vi "CheckFuncInstr.vi"(8 "error in (no error)":errorcluster caption="entrée d'erreur (pas d'erreur)", 11 "Experiment en entrée":refnum<class "Experiment.lvclass"> caption="DNL_LabVIEW Object in") -> (0 "error out":errorcluster caption="sortie d'erreur", 3 "Experiment en sortie":refnum<class "Experiment.lvclass"> caption="DNL_LabVIEW Object out")   [LabVIEW 2019, in "Experiment.lvclass"]
uses:
  Experiment.lvclass
  Experiment.lvclass/Experiment.ctl
  DevicesClass/BaseDevice/BaseDevice.lvclass
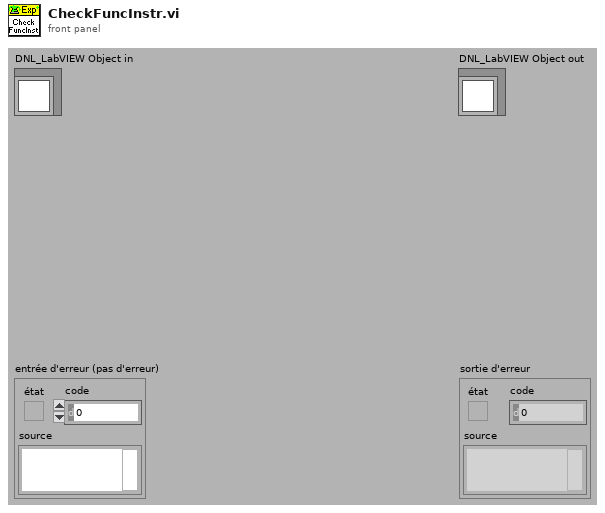
[diagram p1: front panel]
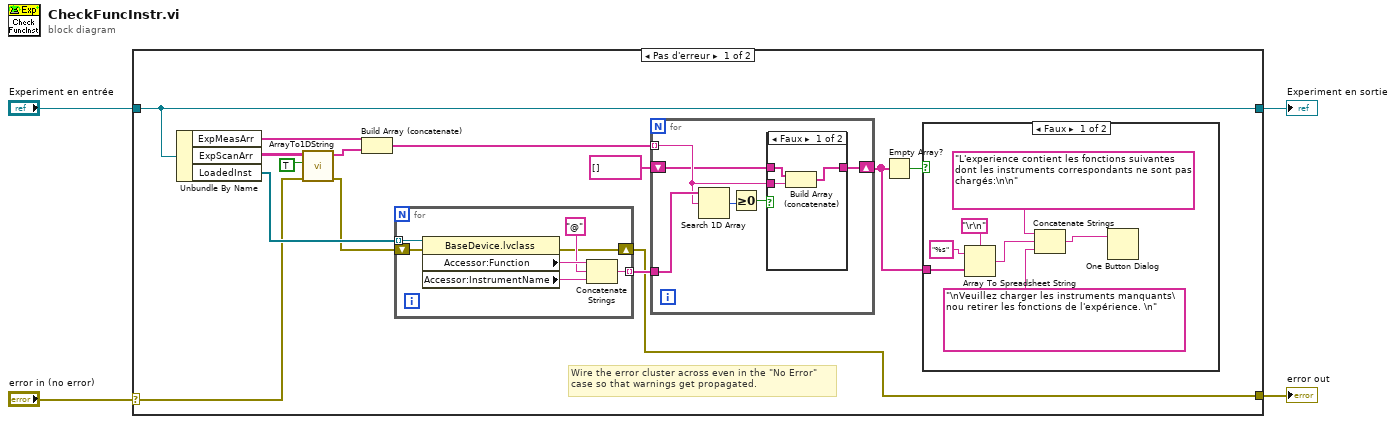
[diagram p0: block diagram]
diagram:
  n1 = case shown="Pas d'erreur" "error in (no error)" {
    selector: "error in (no error)" -> [w10 w44]
    tunnel: [w6 w44] -> w3
    tunnel: [w18 w43] -> w1
    tunnel: "Experiment en entrée" -> [w18 w43]
    frame No Error {
      # "Wire the error cluster across even in the \"No Error\"\ncase so that warnings get propagated."
      n2 = Unbundle By Name(w18) -> ("ExpMeasArr"=w16:string[], "ExpScanArr"=w14:string[][], "LoadedInst"=w17:refnum<class "BaseDevice.lvclass">[])
      n3 = call <userlib>:"ArrayTo1DString.vi"("ErrorIn(No Error)"=w10, "DelArrEnd(F)"=TRUE ("DelArrEnd"), "tableau"=w14) -> ("sortie d'erreur"=w9:errorcluster, "Array Out"=w13:string[])  [unwired: 6 in, 1 out]
      n4 = Build Array (concatenate)(w16, w13) -> (w15:string[])
      n5 = for {
        tunnel: w17 -> [w32] mode=indexing
        tunnel: [w28] -> w11 mode=indexing
        shift-right: [w27] -> w6
        shift-left: w9 -> [w26]
        n6 = property class="BaseDevice.lvclass"(reference=w32, error in=w26) -> (error out=w27:errorcluster, "Accessor:Function"=w31:string, "Accessor:InstrumentName"=w30:string)  [unwired: 1 out]
        n7 = Concatenate Strings(w31, "@" ("chaîne"), w30) -> (w28:string)
      }
      n8 = for {
        tunnel: w15 -> [w34] mode=indexing
        tunnel: w11 -> [w38]
        shift-right: [w35] -> w7
        shift-left: string[] [] -> [w33]
        n9 = Search 1D Array(1D array=w38, element=w34) -> (index of element=w37:i32)  [unwired: 1 in]
        n10 = Greater Or Equal To 0?(x=w37) -> (x >= 0?=w36:bool)
        n11 = case shown="Faux" w36 {
          tunnel: [w40 w42] -> w35
          tunnel: w34 -> [w41 _]
          tunnel: w33 -> [w39 w42]
          frame False {
            n12 = Build Array (concatenate)(w39, w41) -> (w40:string[])
          }
          frame True {
          }
        }
      }
      n13 = Empty Array?(array=w7) -> (empty?=w8:bool)
      n14 = case shown="Faux" w8 {
        tunnel: w7 -> [w25 _]
        frame False {
          n15 = Array To Spreadsheet String(delimiter (Tab)="\r\n", array=w25, 3:"%s" ("séparateur (Tabulation)")) -> (spreadsheet string=w22:string)
          n16 = Concatenate Strings("L'experience contient les fonctions suivantes   dont les instruments correspondants ne sont pas chargés:\n\n", w22, "\nVeuillez charger les instruments manquants\nou retirer les fonctions de l'expérience. \n") -> (w20:string)
          n17 = One Button Dialog(message=w20) -> ()  [unwired: 1 in, 1 out]
        }
        frame True {
        }
      }
    }
    frame Error {
    }
  }
  "error out" <- w3
  "Experiment en sortie" <- w1
